vi "Parse Line Status.vi"(8 "error in (no error)":errorcluster, 10 "Retries (5)":i32=5, 11 "Controller States in":T1) -> (0 "error out":errorcluster, 1 "Power (dBm)":dbl, 2 "Frequency (MHz)":dbl, 3 "Controller States out":T1, 4 "Switch":bool, 5 "Channel":u8)   [LabVIEW 2019, in "Controller.lvlib"]
uses:
  Controller.lvlib
  Controller States.ctl
  <vilib>/regexp/Match Regular Expression.xnode
  <vilib>/ErrorRing/Error Ring.xnode
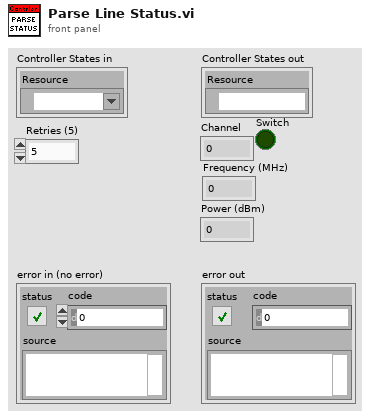
[diagram p1: front panel]
types:
  T1 = typedef "Controller.lvlib/Controller States.ctl" = cluster{"Resource":refnum<visa-resource-name>}
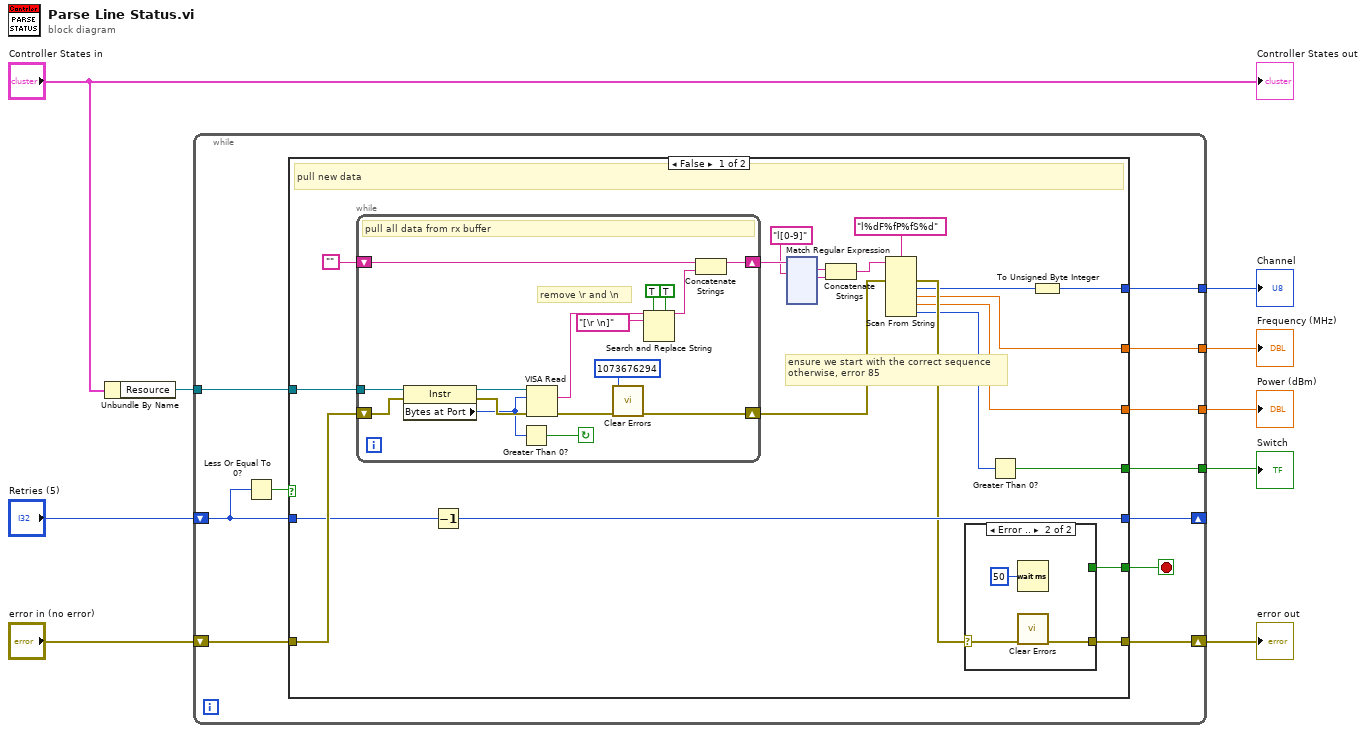
[diagram p0: block diagram]
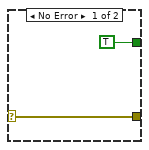
[diagram p2: hidden frame]
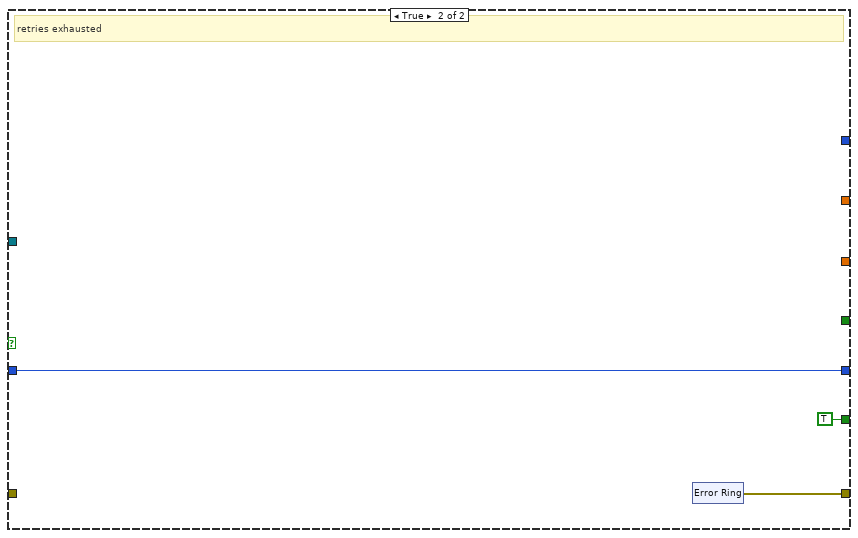
[diagram p3: hidden frame]
diagram:
  n1 = Unbundle By Name("Controller States in") -> ("Resource"=w7:refnum<visa-resource-name>)
  n2 = while {
    tunnel: w7 -> [w19]
    tunnel: [w18] -> w5
    tunnel: [w17] -> w4
    tunnel: [w16] -> w3
    shift-right: [w12] -> w6
    shift-left: "error in (no error)" -> [w20]
    shift-right: [w15] -> _
    shift-left: "Retries (5)" -> [w13]
    tunnel: [w10] -> w1
    stop <- w11 stop-if-true
    n3 = Less Or Equal To 0?(x=w13) -> (x <= 0?=w14:bool)
    n4 = case shown="False" w14 {
      tunnel: w20 -> [w41 _]
      tunnel: w19 -> [w40 _]
      tunnel: [w33 w180] -> w12
      tunnel: [w30 _] -> w10
      tunnel: [w28 _] -> w18
      tunnel: [w27 _] -> w17
      tunnel: [w36 _] -> w16
      tunnel: w13 -> [w35 w181]
      tunnel: [w34 w181] -> w15
      tunnel: [w31 TRUE] -> w11
      frame False {
        # "ensure we start with the correct sequence\notherwise, error 85"
        # "pull new data"
        n5 = while {
          tunnel: w40 -> [w178]
          shift-right: [w171] -> w38
          shift-left: w41 -> [w176]
          shift-right: [w164] -> w25
          shift-left: "" -> [w165]
          stop <- w172 continue-if-true
          # "remove \\r and \\n"
          # "pull all data from rx buffer"
          n6 = property class="Instr"(reference=w178, error in=w176) -> (reference out=w177:refnum<visa-resource-name>, error out=w175:errorcluster, "Bytes at Port"=w173:u32)
          n7 = Greater Than 0?(x=w173) -> (x > 0?=w172:bool)
          n8 = VISA Read(VISA resource name=w177, byte count=w173, error in (no error)=w175) -> (read buffer=w169:string, error out=w174:errorcluster)  [unwired: 2 out]
          n9 = call <vilib>:"Clear Errors.vi"("error in (no error)"=w174, "specific error code to clear (0: all)"=1073676294 ("Code")) -> ("error out"=w171:errorcluster)  [unwired: 4 in, 1 out]
          n10 = Search and Replace String(replace all?=TRUE ("replace all? (F)"), multiline?=TRUE ("multiline? (F)"), input string=w169, search string="[\r \n]") -> (result string=w163:string)  [unwired: 4 in, 3 out]
          n11 = Concatenate Strings(w165, w163) -> (w164:string)
        }
        n12 = Decrement(x=w35) -> (x-1=w34:i32)
        n13 = xnode "Match Regular Expression"("input string"=w25, "regular expression"="l[0-9]") -> ("whole match"=w24:string, "after match"=w23:string)  [unwired: 4 in, 4 out]
        n14 = Concatenate Strings(w24, w23) -> (w22:string)
        n15 = Scan From String(format string="l%dF%fP%fS%d", input string=w22, error in=w38) -> (error out=w32:errorcluster, output 1=w29:i32, output 2=w28:dbl, output 3=w27:dbl, output 4=w26:i32)  [unwired: 5 in, 2 out]
        n16 = case shown="Error .." w32 {
          selector: w32 -> [w159 w162]
          tunnel: [w159 w161] -> w33
          tunnel: [TRUE _] -> w31
          frame No Error {
          }
          frame Error {
            n17 = Wait (ms)(milliseconds to wait=u32 50) -> ()  [unwired: 1 out]
            n18 = call <vilib>:"Clear Errors.vi"("error in (no error)"=w162) -> ("error out"=w161:errorcluster)  [unwired: 5 in, 1 out]
          }
        }
        n19 = Greater Than 0?(x=w26) -> (x > 0?=w36:bool)
        n20 = To Unsigned Byte Integer(number=w29) -> (unsigned 8bit integer=w30:u8)
      }
      frame True {
        # "retries exhausted"
        n21 = xnode "Error Ring"() -> ("error out"=w180:errorcluster)
      }
    }
  }
  "error out" <- w6
  "Channel" <- w1
  "Frequency (MHz)" <- w5
  "Power (dBm)" <- w4
  "Switch" <- w3
  "Controller States out" <- "Controller States in"
